vi "getData.vi"(8 "error in (no error)":errorcluster, 10 "index":u32, 11 "pHandle":u32) -> (0 "error out":errorcluster, 1 "triggerMask":string, 2 "return type":i32, 3 "pData":T1)   [LabVIEW 2011, in "sbgLabView.lvlib"]
uses:
  sbgLabView.lvlib
  sbgMatLab.dll
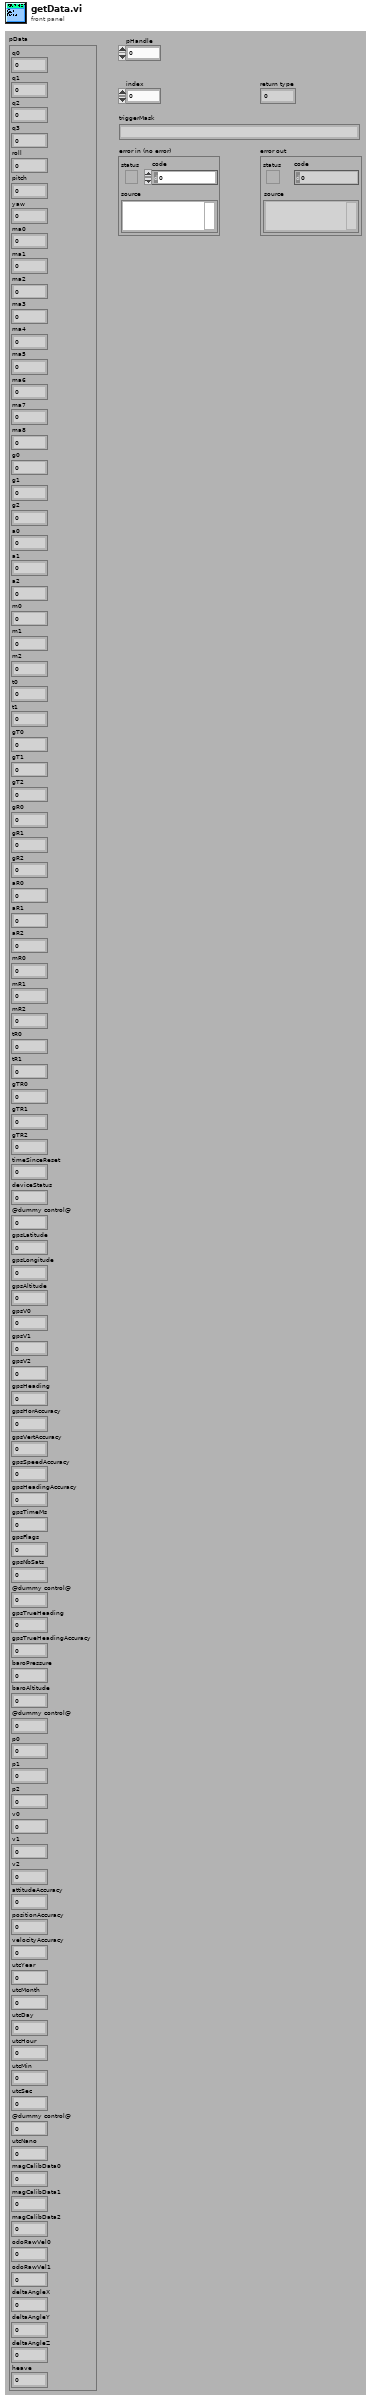
[diagram p1: front panel]
types:
  T1 = cluster{"q0":sgl, "q1":sgl, "q2":sgl, "q3":sgl, "roll":sgl, "pitch":sgl, "yaw":sgl, "ma0":sgl, "ma1":sgl, "ma2":sgl, "ma3":sgl, "ma4":sgl, "ma5":sgl, "ma6":sgl, "ma7":sgl, "ma8":sgl, "g0":sgl, "g1":sgl, "g2":sgl, "a0":sgl, "a1":sgl, "a2":sgl, "m0":sgl, "m1":sgl, "m2":sgl, "t0":sgl, "t1":sgl, "gT0":sgl, "gT1":sgl, "gT2":sgl, "gR0":u16, "gR1":u16, "gR2":u16, "aR0":u16, "aR1":u16, "aR2":u16, "mR0":u16, "mR1":u16, "mR2":u16, "tR0":u16, "tR1":u16, "gTR0":u16, "gTR1":u16, "gTR2":u16, "timeSinceReset":u32, "deviceStatus":sgl, "@dummy control@":u32, "gpsLatitude":dbl, "gpsLongitude":dbl, "gpsAltitude":i32, "gpsV0":i32, "gpsV1":i32, "gpsV2":i32, "gpsHeading":sgl, "gpsHorAccuracy":u32, "gpsVertAccuracy":u32, "gpsSpeedAccuracy":u32, "gpsHeadingAccuracy":sgl, "gpsTimeMs":u32, "gpsFlags":u8, "gpsNbSats":u8, "@dummy control@":u16, "gpsTrueHeading":sgl, "gpsTrueHeadingAccuracy":sgl, "baroPressure":sgl, "baroAltitude":sgl, "@dummy control@":u32, "p0":dbl, "p1":dbl, "p2":dbl, "v0":sgl, "v1":sgl, "v2":sgl, "attitudeAccuracy":sgl, "positionAccuracy":sgl, "velocityAccuracy":sgl, "utcYear":u8, "utcMonth":sgl, "utcDay":sgl, "utcHour":sgl, "utcMin":sgl, "utcSec":u8, "@dummy control@":u16, "utcNano":u32, "magCalibData0":u32, "magCalibData1":u32, "magCalibData2":u32, "odoRawVel0":sgl, "odoRawVel1":sgl, "deltaAngleX":sgl, "deltaAngleY":sgl, "deltaAngleZ":sgl, "heave":sgl}
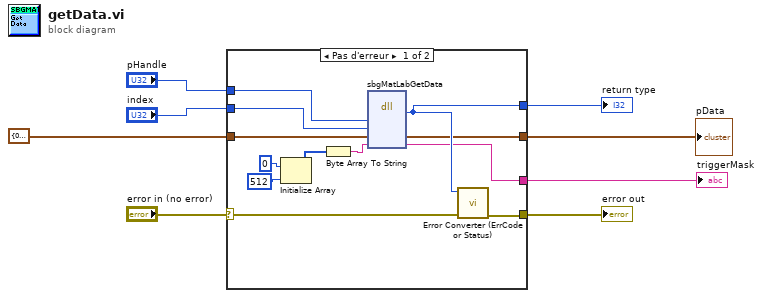
[diagram p0: block diagram]
diagram:
  n1 = case shown="Pas d'erreur" "error in (no error)" {
    selector: "error in (no error)" -> [w17 w22]
    tunnel: [w16 w22] -> w7
    tunnel: [w20 _] -> w6
    tunnel: "pHandle" -> [w19 _]
    tunnel: "index" -> [w18 _]
    tunnel: T1 {"q0"=0.0, "q1"=0.0, "q2"=0.0, "q3"=0.0, "roll"=0.0, "pitch"=0.0, "yaw"=0.0, "ma0"=0.0, "ma1"=0.0, "ma2"=0.0, "ma3"=0.0, "ma4"=0.0, "ma5"=0.0, "ma6"=0.0, "ma7"=0.0, "ma8"=0.0, "g0"=0.0, "g1"=0.0, "g2"=0.0, "a0"=0.0, "a1"=0.0, "a2"=0.0, "m0"=0.0, "m1"=0.0, "m2"=0.0, "t0"=0.0, "t1"=0.0, "gT0"=0.0, "gT1"=0.0, "gT2"=0.0, "gR0"=0, "gR1"=0, "gR2"=0, "aR0"=0, "aR1"=0, "aR2"=0, "mR0"=0, "mR1"=0, "mR2"=0, "tR0"=0, "tR1"=0, "gTR0"=0, "gTR1"=0, "gTR2"=0, "timeSinceReset"=0, "deviceStatus"=0.0, "@dummy control@"=0, "gpsLatitude"=0.0, "gpsLongitude"=0.0, "gpsAltitude"=0, "gpsV0"=0, "gpsV1"=0, "gpsV2"=0, "gpsHeading"=0.0, "gpsHorAccuracy"=0, "gpsVertAccuracy"=0, "gpsSpeedAccuracy"=0, "gpsHeadingAccuracy"=0.0, "gpsTimeMs"=0, "gpsFlags"=0, "gpsNbSats"=0, "@dummy control@"=0, "gpsTrueHeading"=0.0, "gpsTrueHeadingAccuracy"=0.0, "baroPressure"=0.0, "baroAltitude"=0.0, "@dummy control@"=0, "p0"=0.0, "p1"=0.0, "p2"=0.0, "v0"=0.0, "v1"=0.0, "v2"=0.0, "attitudeAccuracy"=0.0, "positionAccuracy"=0.0, "velocityAccuracy"=0.0, "utcYear"=0, "utcMonth"=0.0, "utcDay"=0.0, "utcHour"=0.0, "utcMin"=0.0, "utcSec"=0, "@dummy control@"=0, "utcNano"=0, "magCalibData0"=0, "magCalibData1"=0, "magCalibData2"=0, "odoRawVel0"=0.0, "odoRawVel1"=0.0, "deltaAngleX"=0.0, "deltaAngleY"=0.0, "deltaAngleZ"=0.0, "heave"=0.0} ("pData") -> [w14 w21]
    tunnel: [w15 w21] -> w3
    tunnel: [w13 _] -> w1
    frame No Error {
      n2 = Initialize Array(u8 0 ("element"), 512 ("dimension size")) -> (w12:u8[])
      n3 = Byte Array To String(unsigned byte array=w12) -> (string=w9:string)
      n4 = dll-call lib="C:/SBG-Systems/remote/projects/software/projects/labviewExample/sbgLabView/sbgMatLab.*" fn="sbgMatLabGetData"("pHandle"=w19, "index"=w18, "pData"=w14, "triggerMask"=w9) -> ("return type"=w20:i32, "pData"=w15:T1, "triggerMask"=w13:string)  [unwired: 5 in, 2 out]
      n5 = call "Error Converter (ErrCode or Status).vi"("error in (no error)"=w17, "error code"=w20) -> ("error out"=w16:errorcluster)  [unwired: 9 in]
    }
    frame Error {
    }
  }
  "return type" <- w6
  "error out" <- w7
  "pData" <- w3
  "triggerMask" <- w1
